vi "test Get and Set Transfers.vi"(8 "error in (no error)":errorcluster, 11 "TestCase in":refnum<class "Framework Property Tests.lvclass">) -> (0 "error out":errorcluster, 3 "TestCase out":refnum<class "Framework Property Tests.lvclass">)   [LabVIEW 2017, in "Framework Property Tests.lvclass"]
uses:
  Framework Property Tests.lvclass
  <vilib>/addons/_JKI Toolkits/VI Tester/TestCase.llb/TestCase.lvclass
  Classes/Transfer/Transfer.lvclass
  Classes/Framework/Framework.lvclass
  C:/Program Files (x86)/National Instruments/LabVIEW 2017/vi.lib/addons/_JKI Toolkits/VI Tester/TestCase.llb/TestCase.lvclass
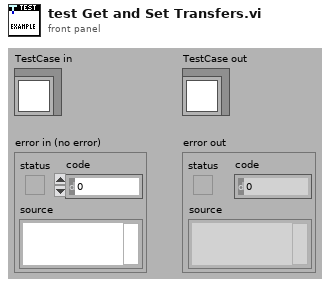
[diagram p1: front panel]
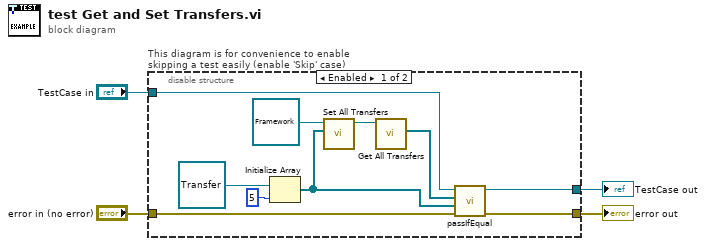
[diagram p0: block diagram]
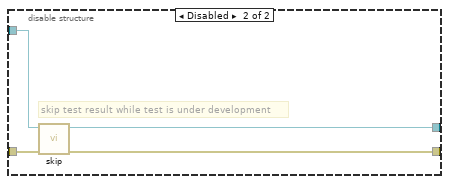
[diagram p2: hidden frame]
diagram:
  n1 = disable-structure "This diagram is for convenience to enable skipping a test easily (enable 'Skip' case)" shown="Enabled" {
    disable-tunnel: "TestCase in" -> [w10 w18]
    disable-tunnel: [w9 w16] -> w1
    disable-tunnel: [w11 w17] -> w3
    disable-tunnel: "error in (no error)" -> [w14 w15]
    frame Enabled {
      n2 = Initialize Array(refnum<class "Transfer.lvclass"> refnum ("Transfers"), 5 ("dimension size")) -> (w8:refnum<class "Transfer.lvclass">[])
      n3 = call "Set All Transfers.vi"("All Transfers"=w8, "Framework in"=refnum<class "Framework.lvclass"> refnum ("Mock Framework in")) -> ("Framework out"=w7:refnum<class "Framework.lvclass">)  [unwired: 9 in]
      n4 = call "Get All Transfers.vi"("Framework in"=w7) -> ("All Transfers"=w6:refnum<class "Transfer.lvclass">[])  [unwired: 9 in, 1 out]
      n5 = call-dynamic "passIfEqual.vi"("error in (no error)"=w14, "y"=w8, "x"=w6, "TestCase in"=w10) -> ("error out"=w11:errorcluster, "TestCase out"=w9:refnum<class "Framework Property Tests.lvclass">)  [unwired: 6 in]
    }
    frame Disabled {
      # "skip test result while test is under development"
      n6 = call <vilib>:"skip.vi"("error in (no error)"=w15, "TestCase in"=w18) -> ("error out"=w17:errorcluster, "TestCase out"=w16:refnum<class "Framework Property Tests.lvclass">)  [unwired: 8 in]
    }
  }
  "error out" <- w3
  "TestCase out" <- w1
